vi "CAD@AddPart(FromFile)__Parameter.vi"(1 "ParamterIn":string) -> (0 "ParamterOut":string)   [LabVIEW 2019]
uses:
  MainFrame/Global.vi
panel:
  in  "Step File":string(combo)
  in  "PartName":string(combo)
  in  "Confirm":bool
  # "CAD@AddPart $PartName,$StepFile"
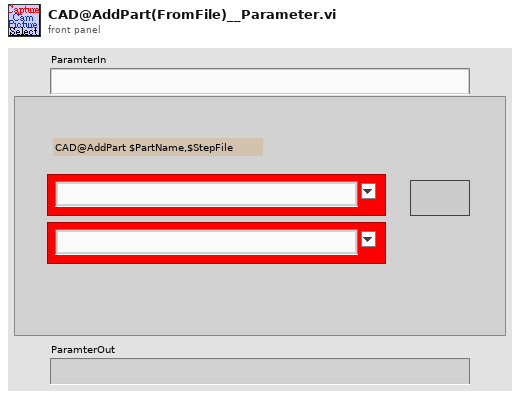
[diagram p1: front panel]
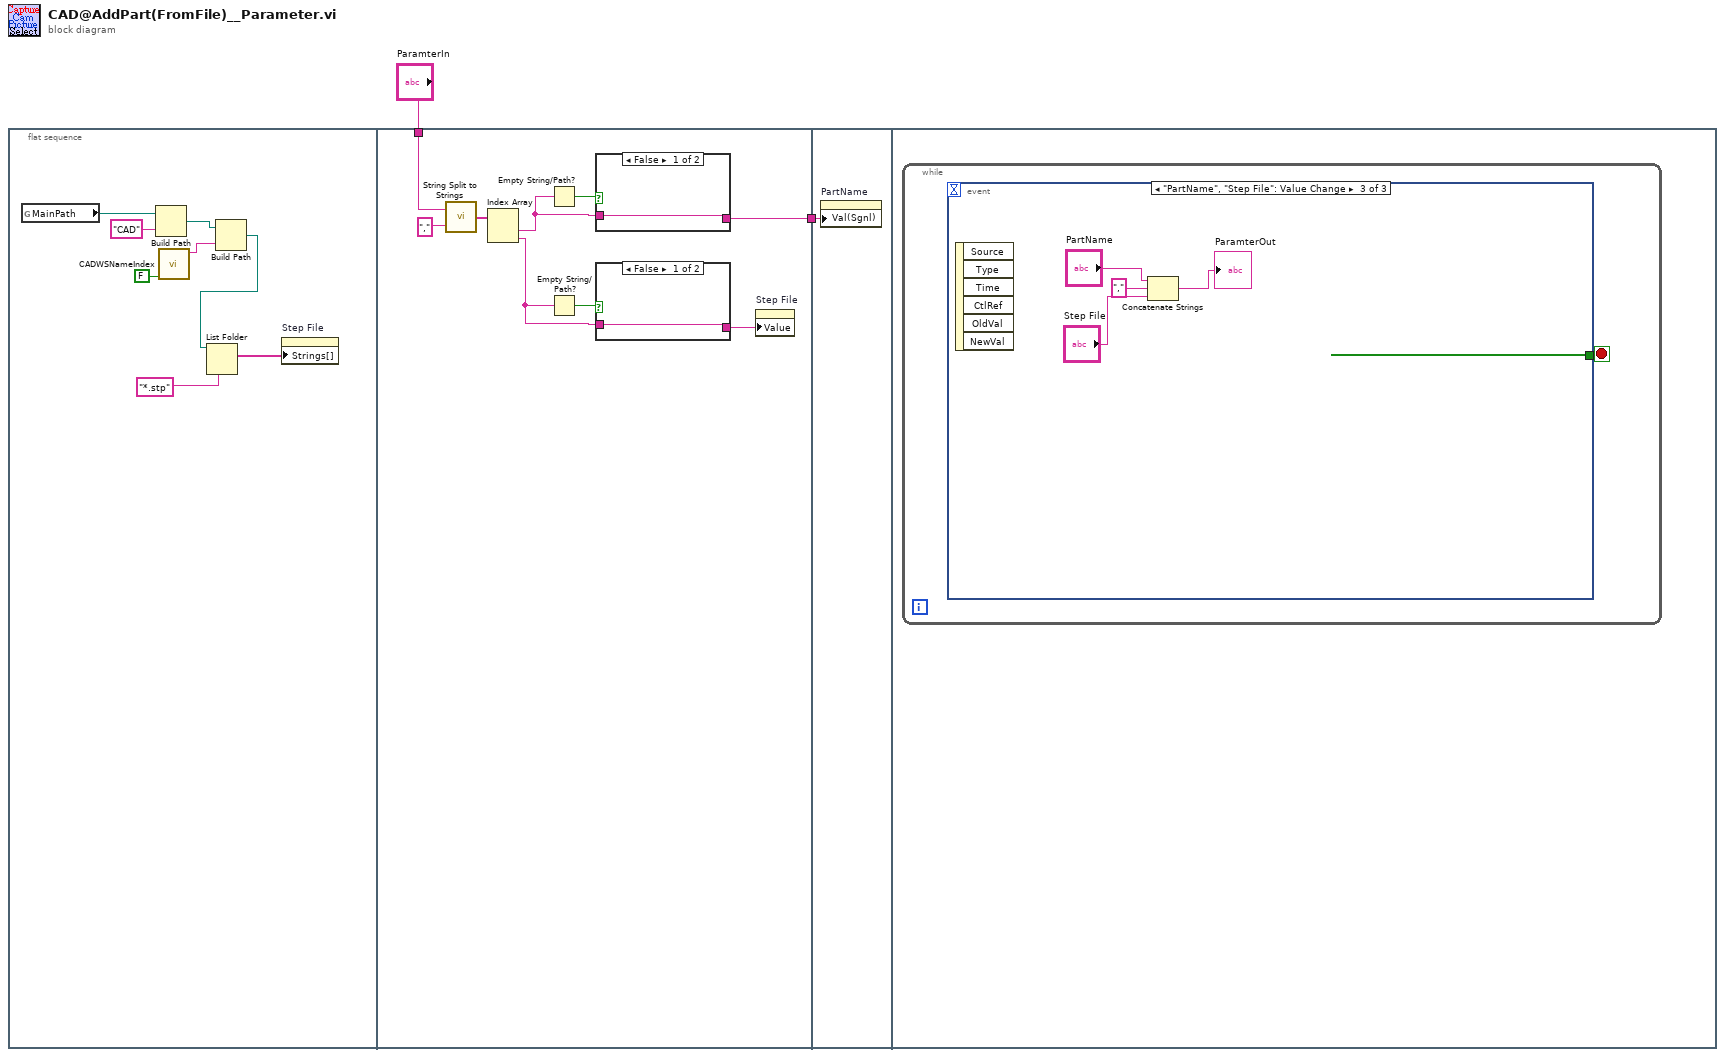
[diagram p0: block diagram]
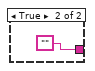
[diagram p2: hidden frame]
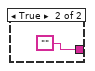
[diagram p3: hidden frame]
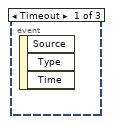
[diagram p4: hidden frame]
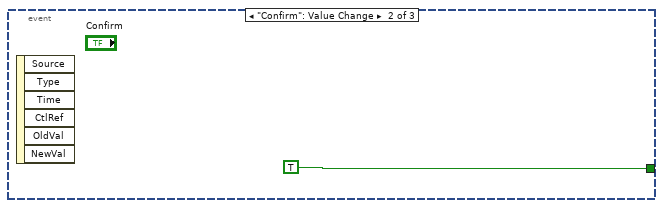
[diagram p5: hidden frame]
diagram:
  n1 = flat-sequence {
    tunnel: "ParamterIn" -> [w17]
    tunnel: [w15] -> w1
    tunnel: w1 -> [w24]
    frame #0 {
      n2 = global read "Global.vi" "MainPath"() -> (w10:path)
      n3 = Build Path(base path=w10, name or relative path="CAD") -> (appended path=w6:path)
      n4 = call "CADWSNameIndex.vi"("Set"=FALSE) -> ("WorkSpaceOut"=w5:string)  [unwired: 10 in]
      n5 = Build Path(base path=w6, name or relative path=w5) -> (appended path=w3:path)
      n6 = List Folder(path=w3, pattern="*.stp") -> (filenames=w7:string[])  [unwired: 2 in, 3 out]
      n7 = property on="Step File" class="CmbBox"("Strings[]"=w7) -> ()  [unwired: 2 in, 2 out]
    }
    frame #1 {
      n8 = call "String Split to Strings.vi"("search string/char (-)"=",", "String"=w17) -> ("Array"=w19:string[])
      n9 = Index Array(array=w19) -> (element #1=w14:string, element #2=w12:string)  [unwired: 2 in]
      n10 = Empty String/Path?(string/path=w14) -> (empty?=w16:bool)
      n11 = Empty String/Path?(string/path=w12) -> (empty?=w13:bool)
      n12 = case shown="False" w16 {
        tunnel: [w22 ""] -> w15
        tunnel: w14 -> [w22 _]
        frame False {
        }
        frame True {
        }
      }
      n13 = case shown="False" w13 {
        tunnel: [w20 ""] -> w11
        tunnel: w12 -> [w20 _]
        frame False {
        }
        frame True {
        }
      }
      n14 = property on="Step File" class="CmbBox"("Value"=w11) -> ()  [unwired: 2 in, 2 out]
    }
    frame #2 {
      n15 = property on="PartName" class="CmbBox"("Val(Sgnl)"=w24) -> ()  [unwired: 2 in, 2 out]
    }
    frame #3 {
      n16 = while {
        stop <- w25 stop-if-true
        n17 = event shown="[2] \"PartName\", \"Step File\": Value Change" {
          selector: _ -> [_ _ _]
          dyn-events: _ -> [_ _ _]
          timeout: _ -> [_ _ _]
          tunnel: [_ TRUE _] -> w25
          event Timeout {
            n18 = event-data() -> ()  [unwired: 1 in, 3 out]
          }
          event "Confirm": Value Change {
            n19 = event-data() -> ()  [unwired: 1 in, 6 out]
          }
          event "PartName", "Step File": Value Change {
            n20 = event-data() -> ()  [unwired: 1 in, 6 out]
            n21 = Concatenate Strings("PartName", "," ("string"), "Step File") -> (→"ParamterOut":string)
          }
        }
      }
    }
  }
